vi "Msg To Queue Actor.vi"(9 "Priority?":bool, 10 "Msg":refnum<class "Msg.lvclass">, 11 "Dev Panel in":refnum<class "Dev Panel.lvclass">) -> (0 "error out":errorcluster)   [LabVIEW 2021, in "Dev Panel.lvclass"]
uses:
  Dev Panel.lvclass
  Actor/Msg/Msg.lvclass
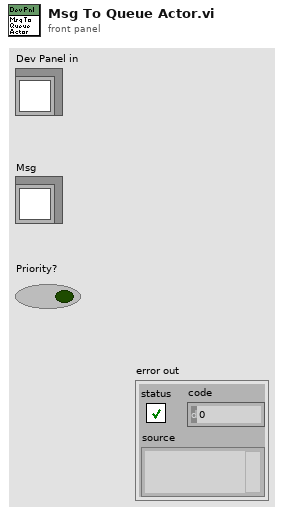
[diagram p1: front panel]
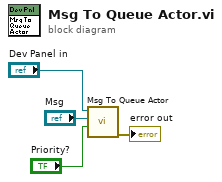
[diagram p0: block diagram]
diagram:
  n1 = call-dynamic "Msg To Queue Actor.vi"("Priority?"="Priority?", "Msg"="Msg", "Dev Panel in"="Dev Panel in") -> ("error out"=→"error out":errorcluster)  [unwired: 8 in]
